vi "ExposeGetObjectMapDefaultValue.vi"(10 "Namepath Data in":T1, 11 "From Value Type":variant) -> (3 "Default Value":variant)   [LabVIEW 2017]
uses:
  ExposeObjectMapNamepathData.ctl
  ExposeObjectMapDataTypeEnum.ctl
  ExposeObjectMapContainerTypeEnum.ctl
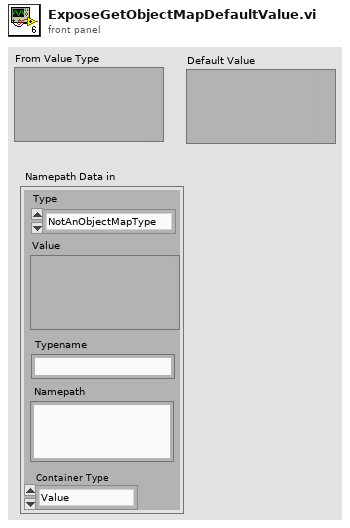
[diagram p1: front panel]
types:
  T1 = typedef "ExposeObjectMapNamepathData.ctl" = cluster{"Type":T2, "Value":variant, "Namepath":string, "Typename":string, "Container Type":T3}
  T2 = typedef "ExposeObjectMapDataTypeEnum.ctl" = enum16{"NotAnObjectMapType", "Real", "Complex", "String", "Boolean"}
  T3 = typedef "ExposeObjectMapContainerTypeEnum.ctl" = enum16{"Value", "Array", "Waveform"}
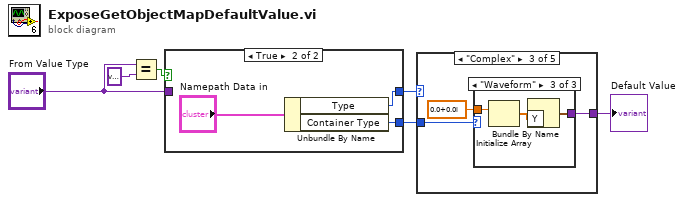
[diagram p0: block diagram]
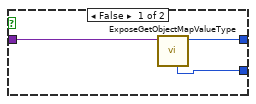
[diagram p2: hidden frame]
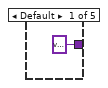
[diagram p3: hidden frame]
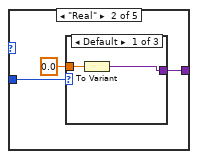
[diagram p4: hidden frame]
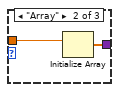
[diagram p5: hidden frame]
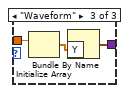
[diagram p6: hidden frame]
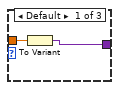
[diagram p7: hidden frame]
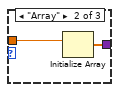
[diagram p8: hidden frame]
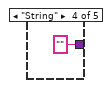
[diagram p9: hidden frame]
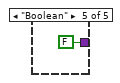
[diagram p10: hidden frame]
diagram:
  n1 = Equal?(x="From Value Type", y=variant) -> (x = y?=w1:bool)
  n2 = case shown="True" w1 {
    tunnel: [w9 w11] -> w6
    tunnel: [w8 w10] -> w4
    tunnel: "From Value Type" -> [w7 _]
    frame False {
      n3 = call "ExposeGetObjectMapValueType.vi"("Value"=w7) -> ("ObjectMapType"=w9:T2, "Container Type (Labview Value type)"=w8:T3)  [unwired: 6 in, 3 out]
    }
    frame True {
      n4 = Unbundle By Name("Namepath Data in") -> ("Type"=w11:T2, "Container Type"=w10:T3)
    }
  }
  n5 = case shown="\"Complex\"" w6 {
    tunnel: [variant w14 w24 "" FALSE] -> w5
    tunnel: w4 -> [_ w16 w26 _ _]
    frame Default {
    }
    frame "Real" {
      n6 = case shown="Default" w16 {
        tunnel: 0.0 -> [w18 w20 w23]
        tunnel: [w17 w19 w21] -> w14
        frame Default {
          n7 = To Variant(anything=w18) -> (Variant=w17:variant)
        }
        frame "Array" {
          n8 = Initialize Array(w20) -> (w19:dbl[])  [unwired: 1 in]
        }
        frame "Waveform" {
          n9 = Initialize Array(w23) -> (w22:dbl[])  [unwired: 1 in]
          n10 = Bundle By Name("Y"=w22) -> (w21:waveform(dbl))  [unwired: 1 in]
        }
      }
    }
    frame "Complex" {
      n11 = case shown="\"Waveform\"" w26 {
        tunnel: cdb 0.0+0.0i -> [w28 w30 w33]
        tunnel: [w27 w29 w31] -> w24
        frame Default {
          n12 = To Variant(anything=w28) -> (Variant=w27:variant)
        }
        frame "Array" {
          n13 = Initialize Array(w30) -> (w29:cdb[])  [unwired: 1 in]
        }
        frame "Waveform" {
          n14 = Initialize Array(w33) -> (w32:cdb[])  [unwired: 1 in]
          n15 = Bundle By Name("Y"=w32) -> (w31:waveform(cdb))  [unwired: 1 in]
        }
      }
    }
    frame "String" {
    }
    frame "Boolean" {
    }
  }
  "Default Value" <- w5
